vi "Write Global Locked.vi"(8 "error in (no error)":errorcluster, 10 "Global":refnum<class "System.lvclass">, 11 "Catapult in":refnum<class "Catapult.lvclass">) -> (0 "error out":errorcluster, 3 "Catapult out":refnum<class "Catapult.lvclass">)   [LabVIEW 2013, in "Catapult.lvclass"]
uses:
  Catapult.lvclass
  System/System.lvclass
  Robot Global Data.vi
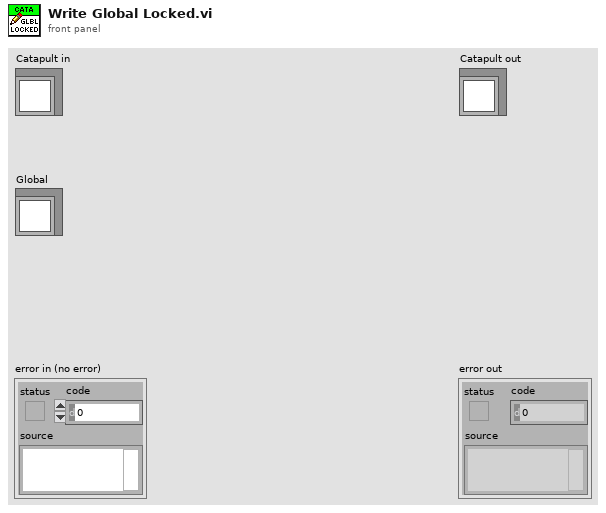
[diagram p1: front panel]
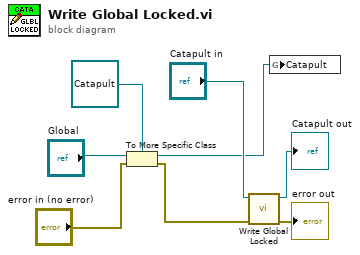
[diagram p0: block diagram]
diagram:
  n1 = To More Specific Class(target class=refnum<class "Catapult.lvclass"> refnum ("Catapult.lvclass"), reference="Global", error in="error in (no error)") -> (specific class reference=w1:refnum<class "Catapult.lvclass">, error out=w2:errorcluster)
  n2 = call-parent "Write Global Locked.vi"("error in (no error)"=w2, "System in"="Catapult in") -> ("error out"=→"error out":errorcluster, "System out"=→"Catapult out":refnum<class "Catapult.lvclass">)  [unwired: 8 in]
  n3 = global write "Robot Global Data.vi" "Catapult"(w1) -> ()
